vi "ESPEC Program Status in Arrsy.vi"(11 "Program State":T1 {"remaining time" format="%<%H:%M>t"}) -> (3 "Program Status":dbl[](array[numeric]))   [LabVIEW 2021, in "Environment Chamber.lvlib"]
uses:
  Environment Chamber.lvlib
  Support Libraries/Climatic Chamber/Private/Type Defs/Program OpState Cluster.ctl
  Support Libraries/Climatic Chamber/Climatic Chamber.lvlib
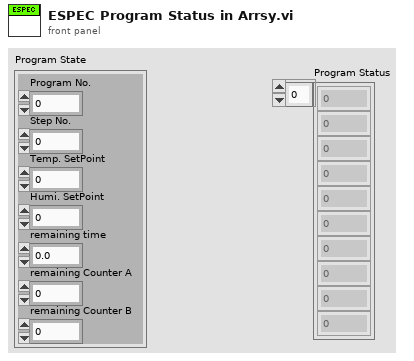
[diagram p1: front panel]
types:
  T1 = typedef "Environment Chamber.lvlib/Climatic Chamber.lvlib/Program OpState Cluster.ctl" = cluster{"Program No.":i32, "Step No.":i32, "Temp. SetPoint":dbl, "Humi. SetPoint":dbl, "remaining time":dbl, "remaining Counter A":i32, "remaining Counter B":i32}
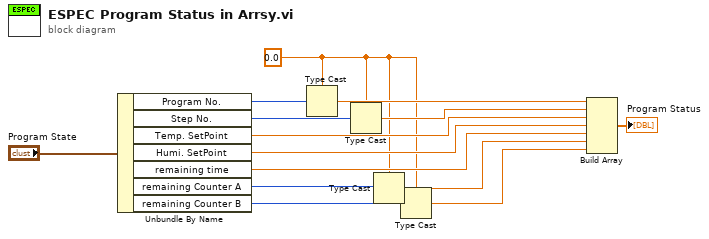
[diagram p0: block diagram]
diagram:
  w3 = 0.0
  n1 = Unbundle By Name("Program State") -> ("Program No."=w13:i32, "Step No."=w12:i32, "Temp. SetPoint"=w9:dbl, "Humi. SetPoint"=w8:dbl, "remaining time"=w7:dbl, "remaining Counter A"=w6:i32, "remaining Counter B"=w4:i32)
  n2 = Type Cast(type=w3, x=w13) -> (*(type *) &x=w11:dbl)
  n3 = Type Cast(type=w3, x=w12) -> (*(type *) &x=w10:dbl)
  n4 = Type Cast(type=w3, x=w6) -> (*(type *) &x=w5:dbl)
  n5 = Type Cast(type=w3, x=w4) -> (*(type *) &x=w2:dbl)
  n6 = Build Array(w11, w10, w9, w8, w7, w5, w2) -> (→"Program Status":dbl[])
